vi "Set Sub Panel Msg.vi"(8 "error in (no error)":errorcluster, 10 "Sub Panel Msg":refnum<vi>, 11 "ENG Actor in":refnum<class "ENG Actor.lvclass">) -> (0 "error out":errorcluster, 3 "ENG Actor out":refnum<class "ENG Actor.lvclass">)   [LabVIEW 2020, in "ENG Actor.lvlib" / "ENG Actor.lvclass"]
uses:
  ENG Actor.lvclass
  ENG Actor.lvclass/ENG Actor.ctl
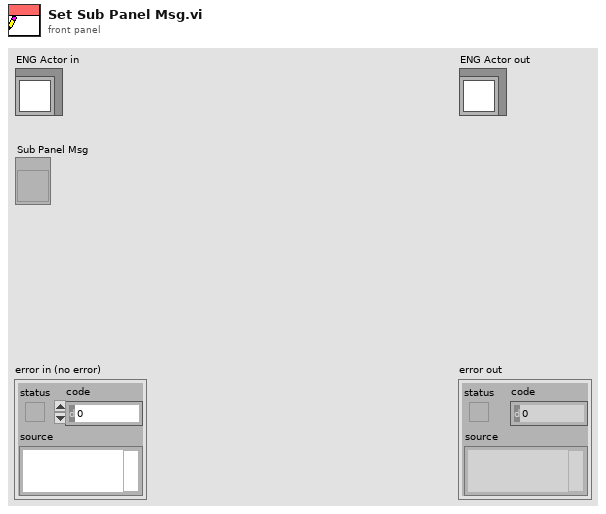
[diagram p1: front panel]
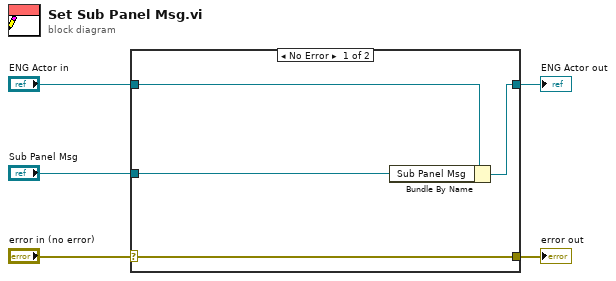
[diagram p0: block diagram]
diagram:
  n1 = case shown="No Error" "error in (no error)" {
    selector: "error in (no error)" -> [w9 w10]
    tunnel: [w9 w10] -> w4
    tunnel: [w7 w11] -> w2
    tunnel: "ENG Actor in" -> [w8 w11]
    tunnel: "Sub Panel Msg" -> [w6 _]
    frame No Error {
      n2 = Bundle By Name(cluster=w8, "Sub Panel Msg"=w6) -> (w7:refnum<class "ENG Actor.lvclass">)
    }
    frame Error {
    }
  }
  "error out" <- w4
  "ENG Actor out" <- w2
